vi "Ultrasonic.vi"() -> ()   [LabVIEW 2020]
uses:
  <vilib>/High Genius/HG_WSI_Tookit/Dependencies/Library/Pulse/Pulse.lvclass
  C:/Program Files (x86)/National Instruments/LabVIEW 2020/vi.lib/High Genius/HG_WSI_Tookit/Dependencies/Library/HG_LIB/HG_LIB.lvclass
  <vilib>/High Genius/HG_WSI_Tookit/Dependencies/Library/ISQ/ISQ.lvclass
  <vilib>/Platform/TimedLoop/XDataNode/timing_clust.ctl
  <vilib>/Platform/TimedLoop/XDataNode/nitl_modes.ctl
  <vilib>/Platform/TimedLoop/XDataNode/wakeup.ctl
  <vilib>/platform/TimedLoop/XDataNode/XDataNode.xnode
  <vilib>/High Genius/HG_WSI_Tookit/Dependencies/Library/HG_LIB/HG_LIB.lvclass
  <vilib>/Platform/TimedLoop/XDataNode/XDNodeRunTimeDep.lvlib
panel:
  out "Numeric":i32
  out "PING":dbl
  in  "Pulse":i32=20 min=0 step=1
  in  "stop":bool
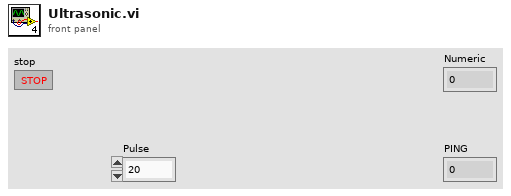
[diagram p1: front panel]
types:
  T1 = enum16{"DI", "DO", "AI", "Pulse", "PWM", "ISQ", "ENC", "CAN", "IIC", "IMU"}
  T2 = enum16{"0", "1", "2", "3", "4", "5", "6", "7", "8", "9", "10", "11", "12", "13", "14", "15", "16", "17", "18", "19", "20", "21", "22", "23", "24", "25"}
  T3 = typedef "XDNodeRunTimeDep.lvlib/timing_clust.ctl" = cluster{"Expected End [f-1]":u64, "Actual End [f-1]":u64, "Finished Late? [f-1]":bool, "Expected End [i-1]":u64, "Actual End [i-1]":u64, "Finished Late? [i-1]":bool, "Expected Start [i]":u64, "Actual Start [i]":u64, "Expected Start [f]":u64, "Actual Start [f]":u64, "Source Name":string, "Structure Name":string, "Period":i64, "Deadline":i64, "Offset":i64, "Start":i64, "Priority":i32, "Timeout":i32, "Mode":T4, "Wakeup Reason":T5, "Error":errorcluster, "Source Type":string, "Secondary Source Type":string, "Global End Time":u64, "Global Start Time":u64, "Frame Duration":u64, "Iteration Duration":u64, "Assigned CPU":i32, "I/O Scan Engine Mode":u32}
  T4 = typedef "XDNodeRunTimeDep.lvlib/nitl_modes.ctl" = enum32{"No Change", "Process missed periods, maintain original phase", "Discard missed periods, maintain original phase", "Process missed periods, ignore original phase", "Discard missed periods, ignore original phase"}
  T5 = typedef "XDNodeRunTimeDep.lvlib/wakeup.ctl" = enum32{"Normal", "Aborted", "Asynchronous wakeup", "Timing source error", "Timed loop error", "Timeout"}
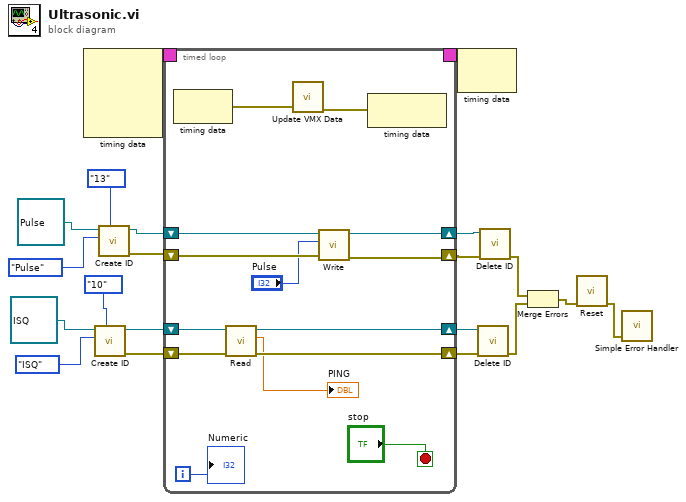
[diagram p0: block diagram]
diagram:
  n1 = node-c288() -> (w20:T3)  [unwired: 4 in]
  n2 = call <vilib>:"Create ID.vi"("NO"=T2."10", "Function"=T1."ISQ", "HG_LIB in"=refnum<class "ISQ.lvclass"> refnum ("VMX Library.lvlib:ISQ.lvclass")) -> ("error out"=w10:errorcluster, "HG_LIB out"=w11:refnum<class "ISQ.lvclass">)  [unwired: 7 in]
  n3 = call <vilib>:"Create ID.vi"("NO"=T2."13", "Function"=T1."Pulse", "HG_LIB in"=refnum<class "Pulse.lvclass"> refnum ("VMX Library.lvlib:Pulse.lvclass")) -> ("error out"=w17:errorcluster, "HG_LIB out"=w13:refnum<class "Pulse.lvclass">)  [unwired: 7 in]
  n4 = timed-loop {
    timing: w20 -> [_]
    timing-out: [_] -> w19
    shift-right: [w30] -> w16
    shift-left: w17 -> [w31]
    shift-right: [w28] -> w12
    shift-left: w13 -> [w29]
    shift-right: [w24] -> w9
    shift-left: w11 -> [w26]
    shift-right: [w23] -> w8
    shift-left: w10 -> [w25]
    i -> [w22]
    stop <- "stop" stop-if-true
    n5 = node-c288() -> (w33:errorcluster)  [unwired: 1 in]
    n6 = call <vilib>:"Read.vi"("error in (no error)"=w25, "ISQ in"=w26) -> ("error out"=w23:errorcluster, "PING"=→"PING":dbl, "ISQ out"=w24:refnum<class "ISQ.lvclass">)  [unwired: 7 in]
    n7 = call <vilib>:"Update VMX Data.vi"("error in (no error)"=w33) -> ("error out"=w32:errorcluster)  [unwired: 10 in]
    n8 = call <vilib>:"Write.vi"("error in (no error)"=w31, "Pulse"="Pulse", "Pulse in"=w29) -> ("error out"=w30:errorcluster, "Pulse out"=w28:refnum<class "Pulse.lvclass">)  [unwired: 7 in]
    n9 = node-c288(w32) -> ()  [unwired: 1 out]
    "Numeric" <- w22
  }
  n10 = node-c288(w19) -> ()  [unwired: 1 out]
  n11 = call <vilib>:"Delete ID.vi"("error in (no error)"=w8, "HG_LIB in"=w9) -> ("error out"=w5:errorcluster)  [unwired: 8 in, 1 out]
  n12 = call <vilib>:"Delete ID.vi"("error in (no error)"=w16, "HG_LIB in"=w12) -> ("error out"=w6:errorcluster)  [unwired: 8 in, 1 out]
  n13 = Merge Errors(w6, w5) -> (w7:errorcluster)
  n14 = call <vilib>:"Reset.vi"("error in (no error)"=w7) -> ("error out"=w18:errorcluster)  [unwired: 10 in]
  n15 = call <vilib>:"Simple Error Handler.vi"("error in (no error)"=w18) -> ()  [unwired: 4 in, 5 out]
